vi "U3 ms Multiple Pulse Output.vi"(8 "error in":errorcluster) -> ()   [LabVIEW 2021]
panel:
  in  "Number of Pulses":dbl=1.0 format="%.2f"
  in  "Pulse Width (ms)":dbl=10.0 min=1.0 max=260.0 step=1.0 format="%.2f"
  in  "FirstFound":bool=TRUE
  in  "Address":string="1"
  out "Error Message":string
  # "Demonstrates using a PWM output and a stop timer to create multiple pulses with a pulse width\nfrom 1-260 ms which is variable in 1 ms increments.  Frequency of the pulses is 3.8 Hz.\n\nThe pulses are negative (signal is normally-high).  If positive pulses are needed, an inverter IC\nshould be put on the signal."
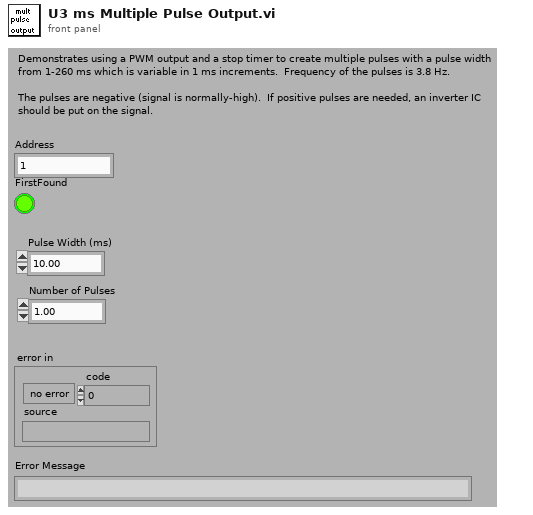
[diagram p1: front panel]
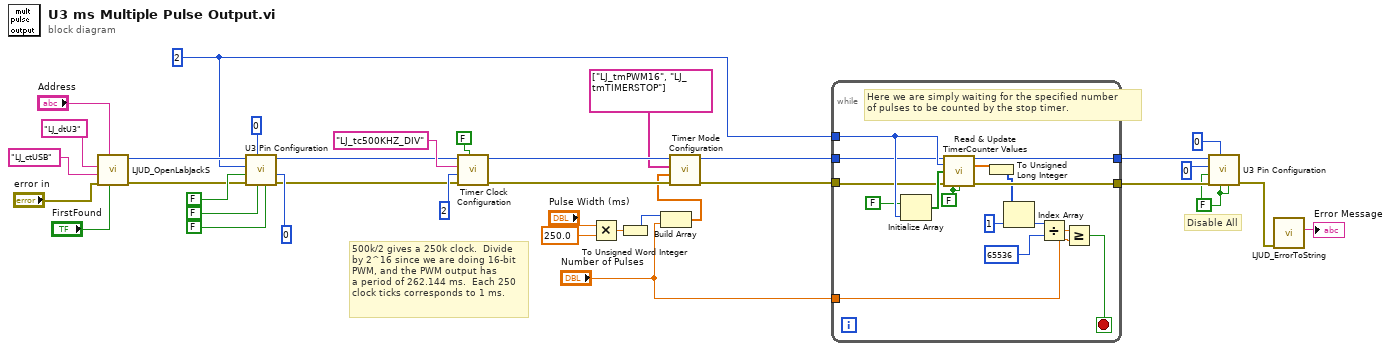
[diagram p0: block diagram]
diagram:
  w1 = FALSE ("Enable Counter0")
  w6 = u8 2 ("Number of Timers Enabled")
  # "Disable All"
  # "500k/2 gives a 250k clock.  Divide\nby 2^16 since we are doing 16-bit\nPWM, and the PWM output has\na period of 262.144 ms.  Each 250\nclock ticks corresponds to 1 ms."
  n1 = call "LJUD_OpenLabJackS.vi"("FirstFound"="FirstFound", "Address"="Address", "error in"="error in", "ConnectionType"="LJ_ctUSB", "DeviceType"="LJ_dtU3") -> ("error out"=w10:errorcluster, "Handle"=w11:i32)  [unwired: 4 in, 1 out]
  n2 = call "U3 Pin Configuration.vi"("Timer/Counter Pin Offset"=u8 0, "Enable Counter1"=FALSE ("Enable Counter0"), "Enable Counter0"=FALSE, "FIO/EIO Analog Enable"=0, "error in"=w10, "Enable DAC1"=FALSE ("Enable Counter0"), "Number of Timers Enabled"=w6, "Handle In"=w11) -> ("error out"=w8:errorcluster, "Handle Out"=w9:i32)  [unwired: 2 in]
  n3 = call "Timer Clock Configuration.vi"("Do Not Do Go()"=FALSE, "error in"=w8, "Timer Clock Divisor"=2, "Timer Clock Base"="LJ_tc500KHZ_DIV", "Handle In"=w9) -> ("error out"=w24:errorcluster, "Handle Out"=w23:i32)  [unwired: 5 in]
  n4 = Multiply(x="Pulse Width (ms)", y=250.0) -> (x*y=w17:dbl)
  n5 = To Unsigned Word Integer(number=w17) -> (unsigned 16bit integer=w14:u16)
  n6 = Build Array(w14, "Number of Pulses") -> (w16:dbl[])
  n7 = call "Timer Mode Configuration.vi"("error in"=w24, "TimerValues"=w16, "TimerModes"=string[] ["LJ_tmPWM16", "LJ_tmTIMERSTOP"], "Handle In"=w23) -> ("error out"=w7:errorcluster, "Handle Out"=w5:i32)  [unwired: 6 in]
  n8 = while {
    tunnel: [w52] -> w4
    tunnel: [w50] -> w32
    tunnel: w6 -> [w49]
    tunnel: w5 -> [w47]
    tunnel: w7 -> [w46]
    tunnel: "Number of Pulses" -> [w37]
    stop <- w39 stop-if-true
    w48 = FALSE ("Reset Counter0")
    # "Here we are simply waiting for the specified number\nof pulses to be counted by the stop timer."
    n9 = Initialize Array(FALSE, w49) -> (w51:bool[])
    n10 = call "Read & Update TimerCounter Values.vi"("Handle In"=w47, "# Timers to Read"=w49, "UpdateReset Timers"=w51, "error in"=w46, "Read Counter0"=w48, "Read Counter1"=w48) -> ("Handle Out"=w50:i32, "Timer Value Reads"=w41:dbl[], "error out"=w52:errorcluster)  [unwired: 6 in, 1 out]
    n11 = To Unsigned Long Integer(number=w41) -> (unsigned 32bit integer=w40:u32[])
    n12 = Index Array(array=w40, index=1 ("Index")) -> (element=w42:u32)
    n13 = Divide(x=w42, y=u32 65536) -> (x/y=w43:dbl)
    n14 = Greater Or Equal?(x=w43, y=w37) -> (x >= y?=w39:bool)
  }
  n15 = call "U3 Pin Configuration.vi"("Enable Counter1"=w1, "Enable Counter0"=w1, "FIO/EIO Analog Enable"=0, "error in"=w4, "Enable DAC1"=w1, "Number of Timers Enabled"=u8 0 ("# Timers Enabled"), "Handle In"=w32) -> ("error out"=w31:errorcluster)  [unwired: 3 in, 1 out]
  n16 = call "LJUD_ErrorToString.vi"("error in"=w31) -> ("String"=→"Error Message":string)  [unwired: 10 in]
